vi "IR_CodeEventExe.vi"(0 "Devices In":u64[](array[numeric]), 1 "Event Registration Refnum In":refnum<event-registration>, 5 "error in (no error)":errorcluster) -> (10 "Index":i32, 12 "Event?":bool, 13 "phid":u64, 14 "Devices Out":u64[](array[numeric]), 15 "Event Registration Refnum Out":refnum<event-registration>, 16 "Code String":string caption="Code", 17 "Bit Count":i32, 18 "Repeat":bool, 19 "error out":errorcluster)   [LabVIEW 2012, in "Phidget IR.lvlib"]
doc: "${Code:Header}"
uses:
  <instrlib>/Phidgets/Phidget IR/Phidget IR.lvlib
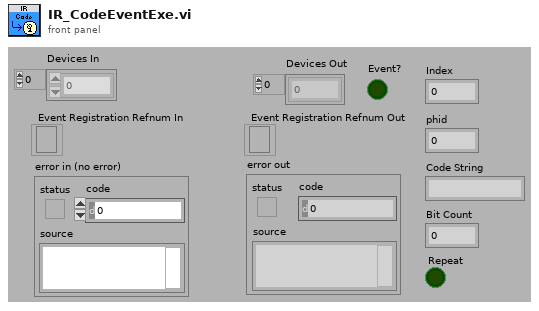
[diagram p1: front panel]
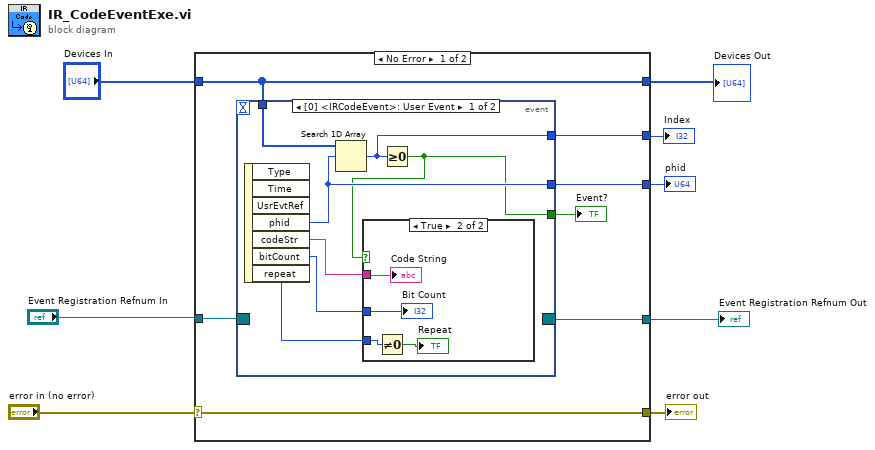
[diagram p0: block diagram]
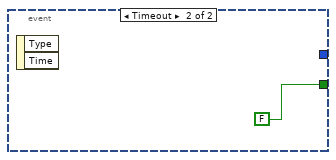
[diagram p3: hidden frame]
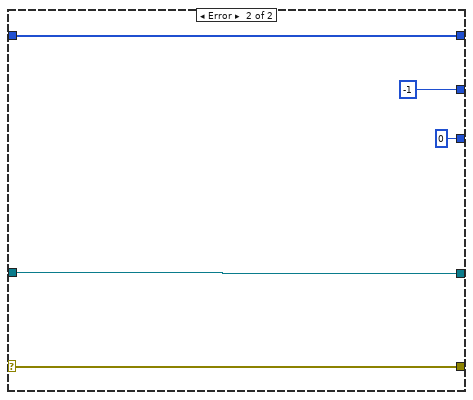
[diagram p4: hidden frame]
diagram:
  n1 = case shown="No Error" "error in (no error)" {
    selector: "error in (no error)" -> [w13 w32]
    tunnel: [w13 w32] -> w7
    tunnel: [w15 w31] -> w1
    tunnel: "Event Registration Refnum In" -> [w14 w31]
    tunnel: [w12 w30] -> w5
    tunnel: "Devices In" -> [w12 w30]
    tunnel: [w11 -1] -> w4
    tunnel: [w10 u64 0 ("phid")] -> w3
    frame No Error {
      n2 = event shown="[0] <IRCodeEvent>: User Event" {
        selector: w14 -> [_ _]
        dyn-events: [_ _] -> w15
        timeout: _ -> [_ _]
        tunnel: w12 -> [w22 _]
        tunnel: [w21 _] -> w11
        tunnel: [w19 _] -> w10
        tunnel: [w18 FALSE] -> w9
        event User Event {
          n3 = event-data() -> ("phid"=w19:u64, "codeStr"=w20:string, "bitCount"=w17:i32, "repeat"=w16:i32)  [unwired: 1 in, 3 out]
          n4 = Search 1D Array(1D array=w22, element=w19) -> (index of element=w21:i32)  [unwired: 1 in]
          n5 = Greater Or Equal To 0?(x=w21) -> (x >= 0?=w18:bool)
          n6 = case shown="True" w18 {
            tunnel: w20 -> [_ w25]
            tunnel: w17 -> [_ w24]
            tunnel: w16 -> [_ w26]
            frame False {
            }
            frame True {
              n7 = Not Equal To 0?(x=w26) -> (x != 0?=→"Repeat":bool)
              "Code String" <- w25
              "Bit Count" <- w24
            }
          }
        }
        event Timeout {
          n8 = event-data() -> ()  [unwired: 1 in, 2 out]
        }
      }
      "Event?" <- w9
    }
    frame Error {
    }
  }
  "error out" <- w7
  "Devices Out" <- w5
  "Index" <- w4
  "phid" <- w3
  "Event Registration Refnum Out" <- w1
